vi "AdbForwardTCP38300.vi"   [LabVIEW 2013]
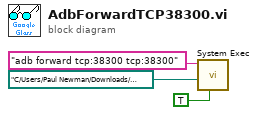
[diagram p0: block diagram]
diagram:
  n1 = call <vilib>:"System Exec.vi"("run minimized? (F)"=TRUE, "working directory"=path "C:/Users/Paul Newman/Downloads/adt-bundle-windows-x86_64-20131030/adt-bundle-windows-x86_64-20131030/sdk", "command line"="adb forward tcp:38300 tcp:38300") -> ()  [unwired: 5 in, 4 out]
